vi "Config Motor.vi"(8 "error in (no error)":errorcluster, 11 "Configuration in":refnum<class "Configuration.lvclass">) -> (0 "error out":errorcluster, 3 "Configuration out":refnum<class "Configuration.lvclass">)   [LabVIEW 2016, in "Hardware.lvlib" / "Motor.lvlib" / "Motor Configuration.lvclass"]
uses:
  <userlib>/Common Components/Hardware/Motor/Motor Config/Motor Configuration.lvclass
  <userlib>/Configuration Dialog Actor/Configuration.lvclass
  <userlib>/Common Components/Hardware/Motor/Motor/Motor_Parameters.ctl
  C:/Program Files (x86)/National Instruments/LabVIEW 2016/user.lib/Configuration Dialog Actor/Configuration.lvclass
  <userlib>/Common Components/Hardware/Motor/Motor Config/Motor Configuration.lvclass/Motor Configuration.ctl
  <userlib>/Common Components/Hardware/Abstract Hardware/Hardware.lvclass/Hardware.ctl
  <userlib>/Common Components/Hardware/Motor/Motor/Motor.lvclass/Motor.ctl
  <userlib>/Common Components/Hardware/DevInfo/DevInfo.lvclass/DevInfo.ctl
  <userlib>/Common Components/Hardware/Abstract Hardware/Read DevInfo.vi
  <userlib>/Common Components/Hardware/DevInfo/Read COMM Address.vi
  <userlib>/Common Components/Hardware/DevInfo/Read Sub-COMM Address.vi
  <userlib>/Common Components/Hardware/DevInfo/Read HW Type.vi
  <userlib>/Common Components/Hardware/DevInfo/Read Device Name.vi
  <userlib>/Common Components/Hardware/Motor/Motor/Motor.lvclass
  C:/Program Files (x86)/National Instruments/LabVIEW 2016/user.lib/Common Components/Hardware/Abstract Hardware/Hardware.lvclass
  <userlib>/Common Components/Hardware/DevInfo/DevInfo.lvclass
panel:
  in  "pos to soft set":dbl
  in  "soft set":bool
  out "Preview Current Pos backend":dbl
  out "Preview Current Pos on Main":dbl
  out "Status":bool
  out "HW Type":string
  out "Sub-COMM Address":string
  out "COMM Address":string
  out "Device Name":string
  in  "motor configurations":T1
  in  "set encoder":bool
  in  "encoder to set":dbl
  in  "Revert":bool
  in  "Apply":bool
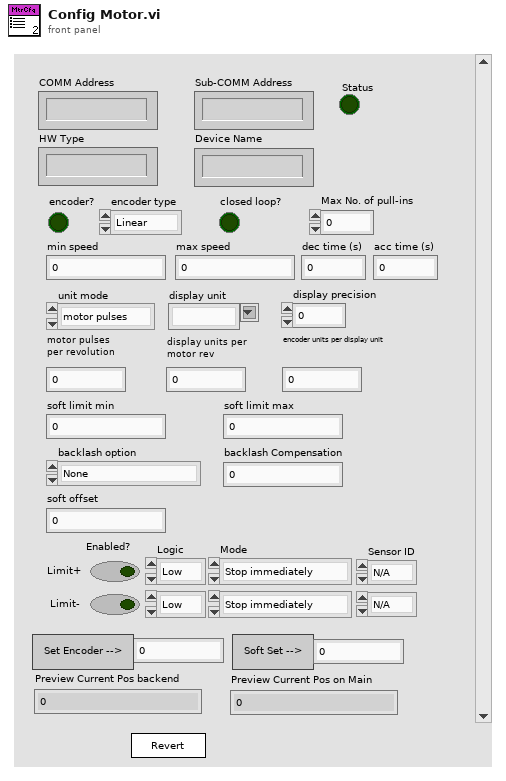
[diagram p1: front panel]
types:
  T1 = typedef "Hardware.lvlib/Motor.lvlib/Motor.lvclass/Motor_Parameters.ctl" = cluster{"closed loop?":bool, "encoder?":bool, "min speed":dbl, "max speed":dbl, "acc time (s)":dbl, "dec time (s)":dbl, "unit mode":enum16{"motor pulses", "real world"}, "motor pulses per revolution":dbl, "display units per motor rev":dbl, "encoder units ratio":dbl, "display unit":string, "display precision":u8, "soft limit min":dbl, "soft limit max":dbl, "Max No. of pull-ins":u8, "Limit+":bool, "Limit+ Logic":enum16{"Low", "High"}, "Limit+ Mode":enum16{"Stop immediately", "Decelerate to Stop"}, "Limit-":bool, "Limit- Logic":enum16{"Low", "High"}, "Limit- Mode":enum16{"Stop immediately", "Decelerate to Stop"}, "Limit+ Sensor ID":enum16{"N/A", "S1", "S2", "S3"}, "Limit- Sensor ID":enum16{"N/A", "S1", "S2", "S3"}, "backlash Compensation":dbl, "soft offset":dbl, "backlash option":enum16{"None", "arriving in + direction", "arriving in - direction"}, "encoder type":enum16{"Linear", "Rotary"}}
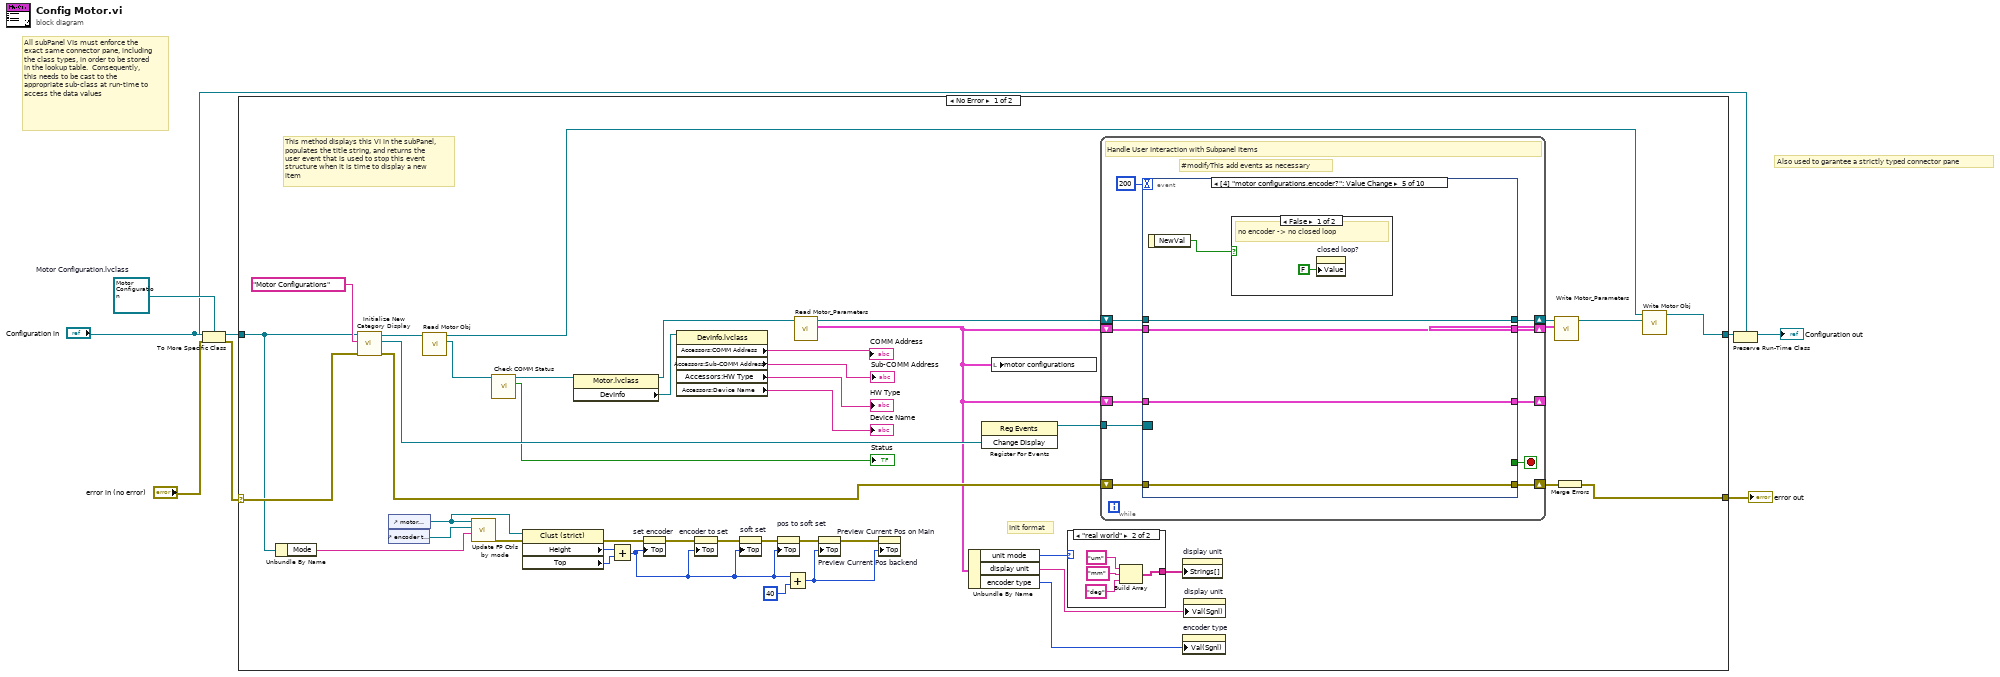
[diagram p0: block diagram]
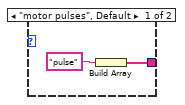
[diagram p2: hidden frame]
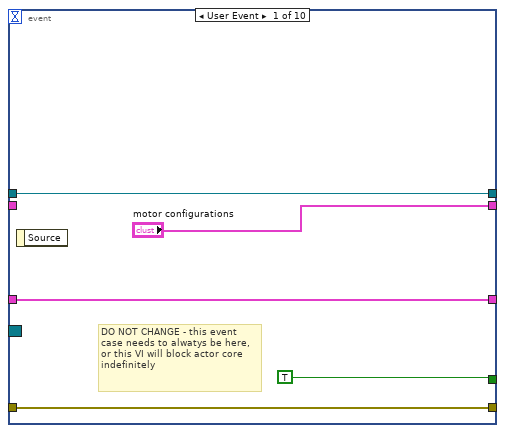
[diagram p3: hidden frame]
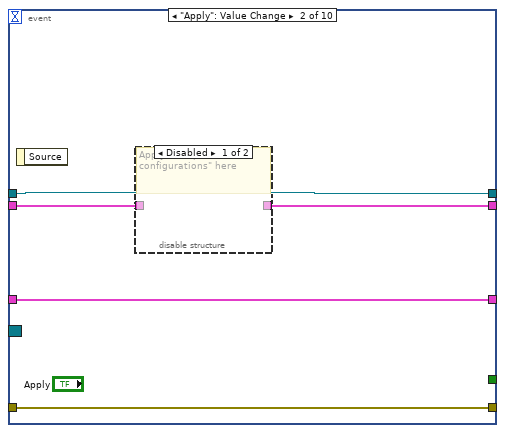
[diagram p4: hidden frame]
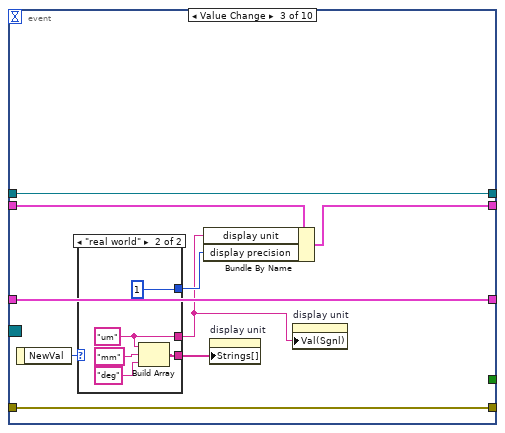
[diagram p6: hidden frame]
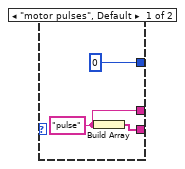
[diagram p7: hidden frame]
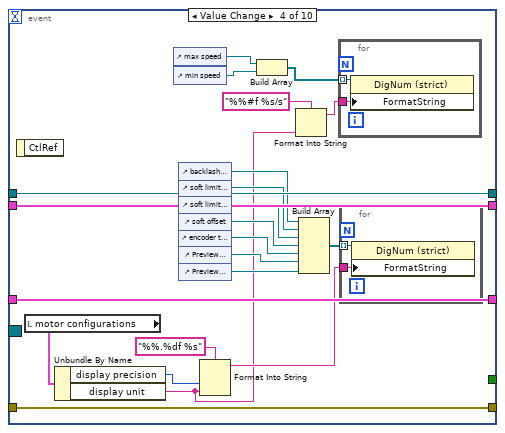
[diagram p8: hidden frame]
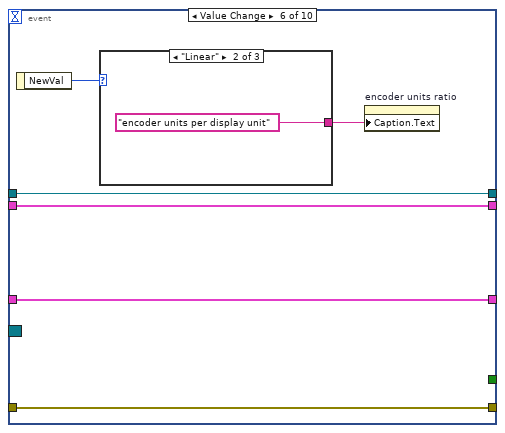
[diagram p10: hidden frame]
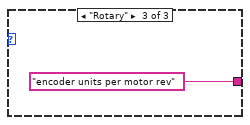
[diagram p12: hidden frame]
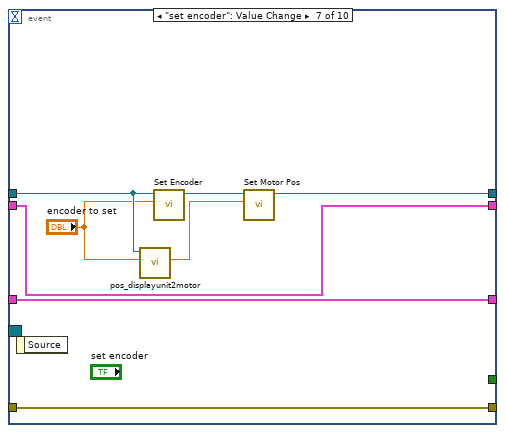
[diagram p13: hidden frame]
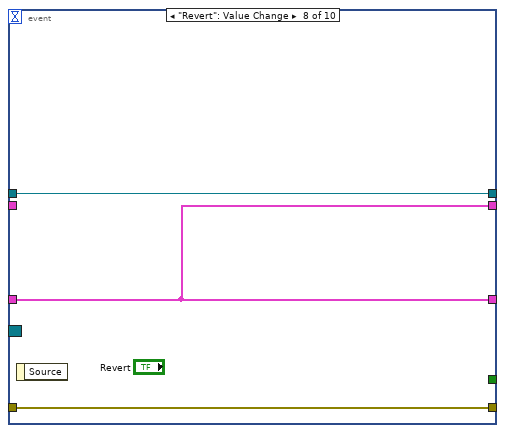
[diagram p14: hidden frame]
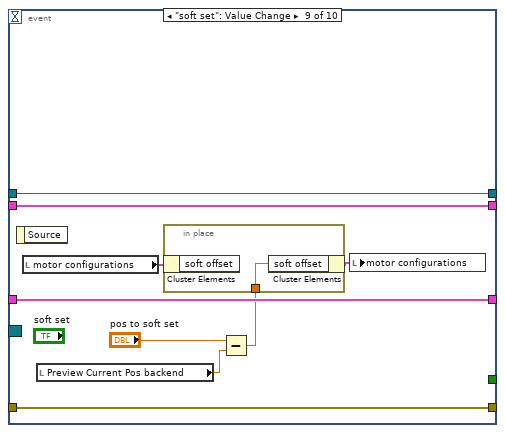
[diagram p15: hidden frame]
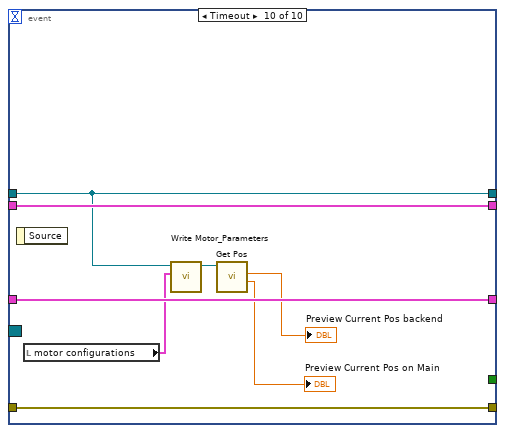
[diagram p16: hidden frame]
diagram:
  w5 = refnum<class "Motor Configuration.lvclass"> refnum  # Motor Configuration.lvclass
  # "Also used to garantee a strictly typed connector pane"
  # "All subPanel VIs must enforce the exact same connector pane, including the class types, in order to be stored in the lookup table.  Consequently, this needs to be cast to the appropriate sub-class at run-time to access the data values"
  n1 = To More Specific Class(target class=w5, reference="Configuration in", error in="error in (no error)") -> (specific class reference=w6:refnum<class "Motor Configuration.lvclass">, error out=w1:errorcluster)
  n2 = case shown="No Error" w1 {
    selector: w1 -> [w48 w167]
    tunnel: w6 -> [w29 w168]
    tunnel: [w38 w168] -> w8
    tunnel: [w50 w167] -> w7
    frame No Error {
      # "Init format"
      # "This method displays this VI in the subPanel, populates the title string, and returns the user event that is used to stop this event structure when it is time to display a new item"
      n3 = Unbundle By Name(w29) -> ("Mode"=w28:string)
      n4 = call <userlib>:"Initialize New Category Display.vi"("error in (no error)"=w48, "Name to Display"="Motor Configurations", "Configuration in"=w29) -> ("error out"=w51:errorcluster, "Change Display"=w47:refnum<user-event>, "Configuration Out"=w52:refnum<class "Motor Configuration.lvclass">)  [unwired: 6 in]
      n5 = control-ref of="motor configurations"() -> (w23:refnum<vi>)
      n6 = control-ref of="encoder to set"() -> (w27:refnum<vi>)
      n7 = call <userlib>:"Read Motor Obj.vi"("Motor Configuration in"=w52) -> ("Hardware.lvlib:Motor.lvlib:Motor.lvclass"=w30:refnum<class "Motor.lvclass">, "Motor Configuration out"=w37:refnum<class "Motor Configuration.lvclass">)  [unwired: 8 in, 1 out]
      n8 = call <userlib>:"Update FP Ctrls by mode.vi"("Mode"=w28, "encoder to set ref"=w27, "motor_parameters ref"=w23) -> ("error out"=w26:errorcluster)  [unwired: 8 in]
      n9 = call-dynamic "Check COMM Status.vi"("Hardware in"=w30) -> ("COMM status"=→"Status":bool, "Hardware out"=w33:refnum<class "Motor.lvclass">)  [unwired: 8 in, 1 out]
      n10 = property class="Clust (strict)"(reference=w23, error in=w26) -> (error out=w24:errorcluster, "Height"=w22:u32, "Top"=w21:i32)  [unwired: 1 out]
      n11 = property class="Motor.lvclass"(reference=w33) -> (reference out=w34:refnum<class "Motor.lvclass">, "DevInfo"=w42:refnum<class "DevInfo.lvclass">)  [unwired: 1 in, 1 out]
      n12 = Add(x=w22, y=w21) -> (x+y=w10:u32)
      n13 = property on="set encoder" class="Bool"(error in=w24, "Top"=w10) -> (error out=w25:errorcluster)  [unwired: 1 in, 1 out]
      n14 = property class="DevInfo.lvclass"(reference=w42) -> ("Accessors:COMM Address"=→"COMM Address":string, "Accessors:Sub-COMM Address"=→"Sub-COMM Address":string, "Accessors:HW Type"=→"HW Type":string, "Accessors:Device Name"=→"Device Name":string)  [unwired: 1 in, 2 out]
      n15 = property on="encoder to set" class="DigNum (strict)"(error in=w25, "Top"=w10) -> (error out=w20:errorcluster)  [unwired: 1 in, 1 out]
      n16 = property on="soft set" class="Bool"(error in=w20, "Top"=w10) -> (error out=w19:errorcluster)  [unwired: 1 in, 1 out]
      n17 = property on="pos to soft set" class="DigNum (strict)"(error in=w19, "Top"=w10) -> (error out=w11:errorcluster)  [unwired: 1 in, 1 out]
      n18 = Add(x=w10, y=u32 40) -> (x+y=w16:u32)
      n19 = call <userlib>:"Read Motor_Parameters.vi"("Motor in"=w34) -> ("motor parameters"=w15:T1, "Motor out"=w36:refnum<class "Motor.lvclass">)  [unwired: 8 in, 1 out]
      n20 = property on="Preview Current Pos backend" class="DigNum (strict)"(error in=w11, "Top"=w16) -> (error out=w18:errorcluster)  [unwired: 1 in, 1 out]
      n21 = property on="Preview Current Pos on Main" class="DigNum (strict)"(error in=w18, "Top"=w16) -> ()  [unwired: 1 in, 2 out]
      n22 = Unbundle By Name(w15) -> ("unit mode"=w14:enum16{"motor pulses", "real world"}, "display unit"=w12:string, "encoder type"=w9:enum16{"Linear", "Rotary"})
      n23 = register-events(w47) -> (reference out=w41:refnum<event-registration>)  [unwired: 2 in, 1 out]
      n24 = local write "motor configurations"(w15) -> ()
      n25 = case shown="\"real world\"" w14 {
        tunnel: [w54 w58] -> w13
        frame "motor pulses", Default {
          n26 = Build Array("pulse") -> (w54:string[])
        }
        frame "real world" {
          n27 = Build Array("um", "mm", "deg") -> (w58:string[])
        }
      }
      n28 = while {
        tunnel: w41 -> [w68]
        shift-right: [w67] -> w39
        shift-left: w15 -> [w66]
        shift-right: [w65] -> _
        shift-left: w15 -> [w64]
        shift-right: [w63] -> w40
        shift-left: w51 -> [w62]
        shift-right: [w60] -> w35
        shift-left: w36 -> [w61]
        stop <- w69 stop-if-true
        # "#modifyThis add events as necessary"
        # "Handle User Interaction with Subpanel Items"
        n29 = event shown="[4] \"motor configurations.encoder?\": Value Change" {
          selector: w68 -> [_ _ _ _ _ _ _ _ _ _]
          dyn-events: _ -> [_ _ _ _ _ _ _ _ _ _]
          timeout: 200 -> [_ _ _ _ _ _ _ _ _ _]
          tunnel: [TRUE _ _ _ _ _ _ _ _ _] -> w69
          tunnel: ["motor configurations" w75 w84 w119 w128 w135 w142 w148 w157 w166] -> w67
          tunnel: w66 -> [_ w76 w85 w119 w128 w135 w142 _ w157 w166]
          tunnel: [w73 w79 w89 w118 w127 w134 w145 w148 w156 w165] -> w65
          tunnel: w64 -> [w73 w79 w89 w118 w127 w134 w145 w148 w156 w165]
          tunnel: [w72 w78 w88 w117 w126 w133 w144 w147 w155 w164] -> w63
          tunnel: w62 -> [w72 w78 w88 w117 w126 w133 w144 w147 w155 w164]
          tunnel: w61 -> [w71 w77 w82 w116 w125 w132 w140 w146 w154 w163]
          tunnel: [w71 w77 w82 w116 w125 w132 w141 w146 w154 w163] -> w60
          event User Event {
            # "DO NOT CHANGE - this event case needs to alwatys be here, or this VI will block actor core indefinitely"
            n30 = event-data() -> ()  [unwired: 1 in, 1 out]
          }
          event "Apply": Value Change {
            n31 = event-data() -> ()  [unwired: 1 in, 1 out]
            n32 = disable-structure shown="Disabled" {
              disable-tunnel: w76 -> [_ w80]
              disable-tunnel: [_ w80] -> w75
              frame Disabled {
                # "Apply new: put \"motor configurations\" here"
              }
              frame Enabled {
              }
            }
          }
          event Value Change {
            n33 = event-data() -> ("NewVal"=w87:enum16{"motor pulses", "real world"})  [unwired: 1 in]
            n34 = case shown="\"real world\"" w87 {
              tunnel: [w92 w97] -> w86
              tunnel: [w91 w95] -> w81
              tunnel: [0 1] -> w83
              frame "motor pulses", Default {
                w91 = "pulse"
                n35 = Build Array(w91) -> (w92:string[])
              }
              frame "real world" {
                w95 = "um"
                n36 = Build Array(w95, "mm", "deg") -> (w97:string[])
              }
            }
            n37 = Bundle By Name(cluster=w85, "display unit"=w81, "display precision"=w83) -> (w84:T1)
            n38 = property on="display unit" class="CmbBox"("Strings[]"=w86) -> ()  [unwired: 2 in, 2 out]
            n39 = property on="display unit" class="CmbBox"("Val(Sgnl)"=w81) -> ()  [unwired: 2 in, 2 out]
          }
          event Value Change {
            n40 = event-data() -> ()  [unwired: 1 in, 1 out]
            n41 = local read "motor configurations"() -> (w115:T1)
            n42 = Unbundle By Name(w115) -> ("display precision"=w113:u8, "display unit"=w100:string)
            n43 = control-ref of="max speed"() -> (w103:refnum<vi>)
            n44 = control-ref of="min speed"() -> (w102:refnum<vi>)
            n45 = control-ref of="backlash Compensation"() -> (w110:refnum<vi>)
            n46 = control-ref of="soft limit max"() -> (w109:refnum<vi>)
            n47 = control-ref of="soft limit min"() -> (w108:refnum<vi>)
            n48 = control-ref of="soft offset"() -> (w107:refnum<vi>)
            n49 = control-ref of="encoder to set"() -> (w104:refnum<vi>)
            n50 = control-ref of="Preview Current Pos backend"() -> (w106:refnum<vi>)
            n51 = control-ref of="Preview Current Pos on Main"() -> (w105:refnum<vi>)
            n52 = Format Into String(format string="%%.%df %s" ("Format String"), w113, w100) -> (resulting string=w111:string)  [unwired: 2 in, 1 out]
            n53 = Build Array(w103, w102) -> (w101:refnum<vi>[])
            n54 = Format Into String(format string="%%#f %s/s" ("Format String"), w100) -> (resulting string=w99:string)  [unwired: 2 in, 1 out]
            n55 = Build Array(w110, w109, w108, w107, w104, w106, w105) -> (w112:refnum<vi>[])
            n56 = for {
              tunnel: w101 -> [w121] mode=indexing
              tunnel: w99 -> [w120]
              n57 = property class="DigNum (strict)"(reference=w121, "FormatString"=w120) -> ()  [unwired: 1 in, 2 out]
            }
            n58 = for {
              tunnel: w112 -> [w123] mode=indexing
              tunnel: w111 -> [w122]
              n59 = property class="DigNum (strict)"(reference=w123, "FormatString"=w122) -> ()  [unwired: 1 in, 2 out]
            }
          }
          event Value Change {
            n60 = event-data() -> ("NewVal"=w124:bool)  [unwired: 1 in]
            n61 = case shown="False" w124 {
              frame False {
                # "no encoder -> no closed loop"
                n62 = property on="closed loop?" class="Bool (strict)"("Value"=FALSE) -> ()  [unwired: 2 in, 2 out]
              }
              frame True {
              }
            }
          }
          event Value Change {
            n63 = event-data() -> ("NewVal"=w131:enum16{"Linear", "Rotary"})  [unwired: 1 in]
            n64 = case shown="\"Linear\"" w131 {
              tunnel: [_ "encoder units per display unit" "encoder units per motor rev"] -> w130
              frame Default {
              }
              frame "Linear" {
              }
              frame "Rotary" {
              }
            }
            n65 = property on="encoder units ratio" class="DigNum (strict)"("Caption.Text"=w130) -> ()  [unwired: 2 in, 2 out]
          }
          event "set encoder": Value Change {
            n66 = event-data() -> ()  [unwired: 1 in, 1 out]
            n67 = call <userlib>:"pos_displayunit2motor.vi"("pos in display unit"="encoder to set", "Motor in"=w140) -> ("pos in motor (pulses)"=w138:dbl)  [unwired: 7 in, 2 out]
            n68 = call <userlib>:"Set Encoder.vi"("encoder pos in display unit"="encoder to set", "Motor in"=w140) -> ("Motor out"=w143:refnum<class "Motor.lvclass">)  [unwired: 8 in, 1 out]
            n69 = call-dynamic "Set Motor Pos.vi"("motor pos (pulse)"=w138, "Motor in"=w143) -> ("Motor out"=w141:refnum<class "Motor.lvclass">)  [unwired: 8 in, 1 out]
          }
          event "Revert": Value Change {
            n70 = event-data() -> ()  [unwired: 1 in, 1 out]
          }
          event "soft set": Value Change {
            n71 = event-data() -> ()  [unwired: 1 in, 1 out]
            n72 = local read "motor configurations"() -> (w153:T1)
            n73 = local read "Preview Current Pos backend"() -> (w150:dbl)
            n74 = Subtract(x="pos to soft set", y=w150) -> (x-y=w149:dbl)
            n75 = in-place {
              in-place-border: w149 -> [w158]
              n76 = in-place-cluster #1(w153) -> ()  [unwired: 1 out]
              n77 = in-place-cluster #1("soft offset"=w158) -> (w152:T1)
            }
            n78 = local write "motor configurations"(w152) -> ()
          }
          event Timeout {
            n79 = event-data() -> ()  [unwired: 1 in, 1 out]
            n80 = local read "motor configurations"() -> (w162:T1)
            n81 = call <userlib>:"Write Motor_Parameters.vi"("motor parameters"=w162, "Motor in"=w163) -> ("Motor out"=w161:refnum<class "Motor.lvclass">)  [unwired: 8 in, 1 out]
            n82 = call <userlib>:"Get Pos.vi"("Motor in"=w161) -> ("Position in display unit (frontend)"=→"Preview Current Pos on Main":dbl, "Position in display unit (backend)"=→"Preview Current Pos backend":dbl)  [unwired: 7 in, 2 out]
          }
        }
      }
      n83 = property on="display unit" class="CmbBox"("Strings[]"=w13) -> ()  [unwired: 2 in, 2 out]
      n84 = property on="encoder type" class="Enum (strict)"("Val(Sgnl)"=w9) -> ()  [unwired: 2 in, 2 out]
      n85 = property on="display unit" class="CmbBox"("Val(Sgnl)"=w12) -> ()  [unwired: 2 in, 2 out]
      n86 = call <userlib>:"Write Motor_Parameters.vi"("motor parameters"=w39, "Motor in"=w35) -> ("Motor out"=w31:refnum<class "Motor.lvclass">)  [unwired: 8 in, 1 out]
      n87 = Merge Errors(w40) -> (w50:errorcluster)
      n88 = call <userlib>:"Write Motor Obj.vi"("Hardware.lvlib:Motor.lvlib:Motor.lvclass"=w31, "Motor Configuration in"=w37) -> ("Motor Configuration out"=w38:refnum<class "Motor Configuration.lvclass">)  [unwired: 8 in, 1 out]
    }
    frame Error {
    }
  }
  "error out" <- w7
  n89 = Preserve Run-Time Class(object in=w8, 2:"Configuration in") -> (object out=→"Configuration out":refnum<class "Configuration.lvclass">)  [unwired: 1 in, 1 out]
